vi "reference global variable 2.vi"() -> ()   [LabVIEW 2015]
panel:
  out "Boolean":bool
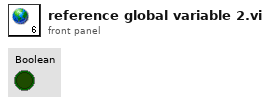
[diagram p1: front panel]
diagram:
